vi "MultiCams.vi"() -> ()   [LabVIEW 2023]
uses:
  <vilib>/userDefined/High Color/IMAQdx.ctl
  <resource>/objmgr/imaqdx.rc
panel:
  in  "Fill in":bool
  in  "OK Button":bool
  in  "CamsToken":string caption="File name"
  in  "CamsDirectory":path caption="Directory"
  out "error out":errorcluster
  in  "Stop":bool
  in  "Camera":T1
  in  "Launch":bool
  in  "Stop and close":bool
  # "Launcher"
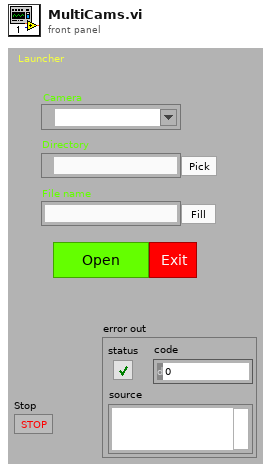
[diagram p1: front panel]
types:
  T1 = typedef "IMAQdx.ctl" = refnum<k21>
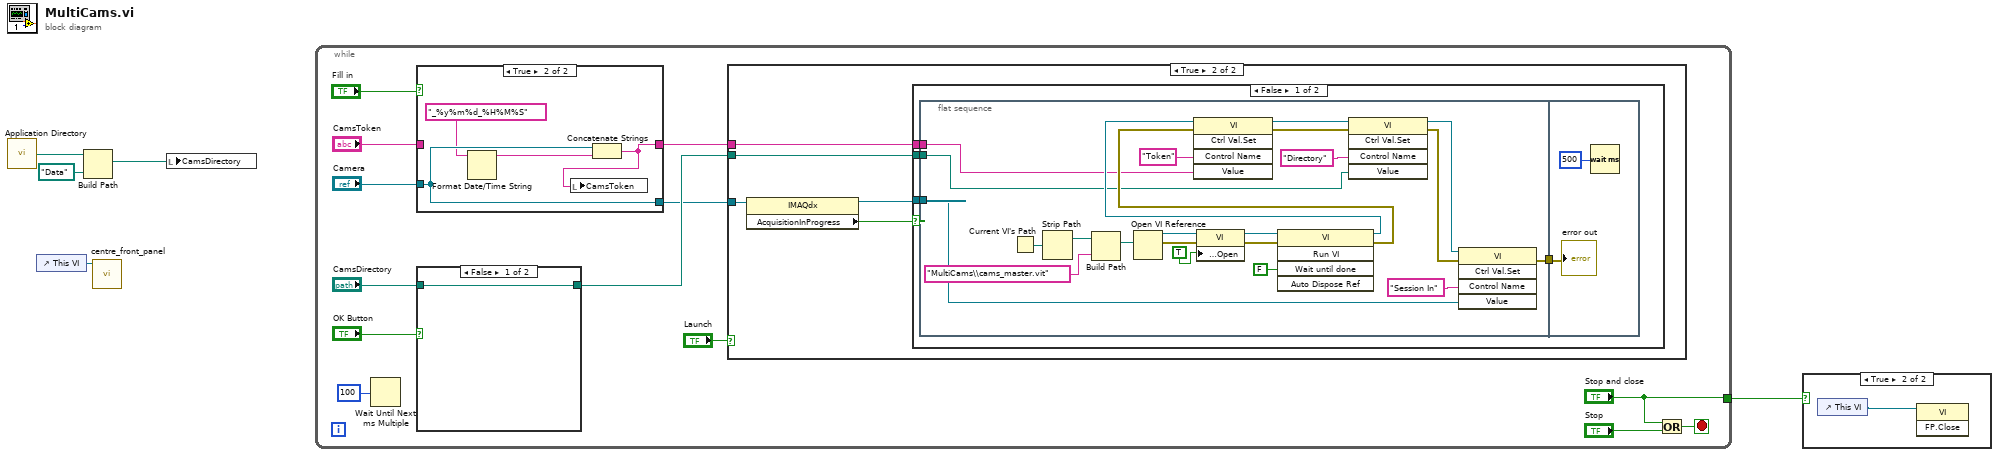
[diagram p0: block diagram]
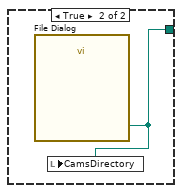
[diagram p4: hidden frame]
diagram:
  n1 = call <vilib>:"Application Directory.vi"() -> ("Application Directory"=w1:path)
  n2 = control-ref of="This VI"() -> (w4:refnum<vi>)
  n3 = Build Path(base path=w1, name or relative path=path "Data") -> (appended path=w3:path)
  n4 = call "centre_front_panel.vi"("VI in"=w4) -> ()  [unwired: 11 in]
  n5 = local write "CamsDirectory"(w3) -> ()
  n6 = while {
    tunnel: ["Stop and close"] -> w5
    stop <- w16 stop-if-true
    n7 = Wait Until Next ms Multiple(millisecond multiple=u32 100) -> ()  [unwired: 1 out]
    n8 = case shown="True" "Fill in" {
      tunnel: [w19 w21] -> w6
      tunnel: "CamsToken" -> [w19 _]
      tunnel: [w20 w23] -> w8
      tunnel: "Camera" -> [w20 w23]
      frame False {
      }
      frame True {
        n9 = Format Date/Time String(time format string (%c)="_%y%m%d_%H%M%S") -> (date/time string=w24:string)  [unwired: 2 out]
        n10 = Concatenate Strings(w23, w24) -> (w21:string)
        n11 = local write "CamsToken"(w21) -> ()
      }
    }
    n12 = case shown="False" "OK Button" {
      tunnel: [w25 w26] -> w11
      tunnel: "CamsDirectory" -> [w25 _]
      frame False {
      }
      frame True {
        n13 = call "File Dialog"() -> ("selected path"=w26:path)  [unwired: 12 in, 3 out]
        n14 = local write "CamsDirectory"(w26) -> ()
      }
    }
    n15 = case shown="True" "Launch" {
      tunnel: w11 -> [_ w29]
      tunnel: w8 -> [_ w28]
      tunnel: w6 -> [_ w27]
      frame False {
      }
      frame True {
        n16 = property class="IMAQdx"(reference=w28) -> (reference out=w30:T1, "AcquisitionInProgress"=w31:bool)  [unwired: 1 in, 1 out]
        n17 = case shown="False" w31 {
          tunnel: w30 -> [w35 _]
          tunnel: w29 -> [w33 _]
          tunnel: w27 -> [w32 _]
          frame False {
            n18 = flat-sequence {
              tunnel: w35 -> [w46]
              tunnel: [w58] -> w34
              tunnel: w33 -> [w37]
              tunnel: w32 -> [w36]
              tunnel: w34 -> [w59]
              frame #0 {
                n19 = Current VI's Path() -> (path=w54:path)
                n20 = Strip Path(path=w54) -> (stripped path=w55:path)  [unwired: 1 out]
                n21 = Build Path(base path=w55, name or relative path="MultiCams\\cams_master.vit") -> (appended path=w56:path)
                n22 = Open VI Reference(vi path=w56) -> (vi reference=w50:refnum<vi>, error out=w52:errorcluster)  [unwired: 5 in]
                n23 = property on="Property Node" class="VI"(reference=w50, error in=w52, "Front Panel Window:Open"=TRUE) -> (reference out=w51:refnum<vi>, error out=w53:errorcluster)
                n24 = invoke class="VI" method="Run VI"(reference=w51, error in=w53, "Wait until done"=FALSE) -> (reference out=w45:refnum<vi>, error out=w44:errorcluster)  [unwired: 2 in, 3 out]
                n25 = invoke class="VI" method="Ctrl Val.Set"(reference=w45, error in=w44, "Control Name"="Token", "Value"=w36) -> (reference out=w43:refnum<vi>, error out=w42:errorcluster)  [unwired: 1 in, 3 out]
                n26 = invoke class="VI" method="Ctrl Val.Set"(reference=w43, error in=w42, "Control Name"="Directory", "Value"=w37) -> (reference out=w41:refnum<vi>, error out=w40:errorcluster)  [unwired: 1 in, 3 out]
                n27 = invoke class="VI" method="Ctrl Val.Set"(reference=w41, error in=w40, "Control Name"="Session In", "Value"=w46) -> (error out=w58:errorcluster)  [unwired: 1 in, 4 out]
              }
              frame #1 {
                n28 = Wait (ms)(milliseconds to wait=u32 500) -> ()  [unwired: 1 out]
                "error out" <- w59
              }
            }
          }
          frame True {
          }
        }
      }
    }
    n29 = Or(x="Stop and close", y="Stop") -> (x .or. y?=w16:bool)
  }
  n30 = case shown="True" w5 {
    frame False {
    }
    frame True {
      n31 = control-ref of="This VI"() -> (w61:refnum<vi>)
      n32 = invoke class="VI" method="FP.Close"(reference=w61) -> ()  [unwired: 2 in, 3 out]
    }
  }
